vi "CreateTemporaryPath.vi"(8 "error in (no error)":errorcluster, 10 "InitalValue":T1, 11 "object in":refnum<class "Crypter.lvclass">) -> (0 "error out":errorcluster, 2 "ReferenceVariableOut":refnum<data-value>, 3 "object out":refnum<class "Crypter.lvclass">)   [LabVIEW 2018]
doc: "This VI creates a DVR reference for a variable."
uses:
  Crypter.lvclass
  C:/Users/Marco Preziani/Documents/Help_Crypting_repository/WebBrowser_Mgmt/WebBrowser_Mgmt.lvclass
  TemporaryPath.ctl
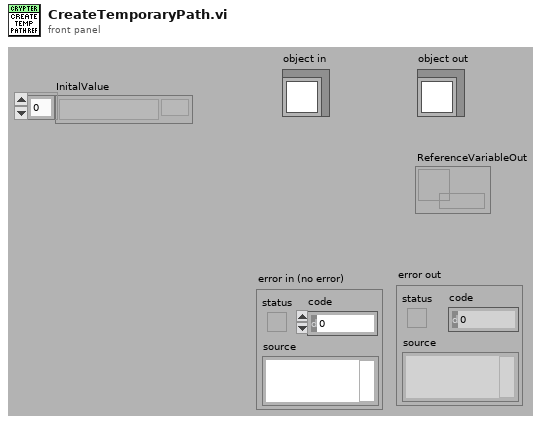
[diagram p1: front panel]
types:
  T1 = typedef "TemporaryPath.ctl" = path[]
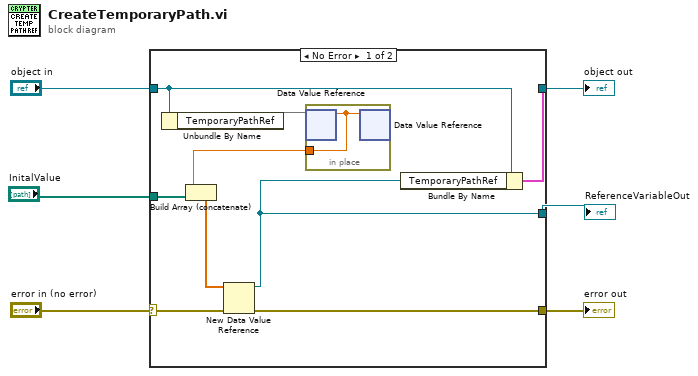
[diagram p0: block diagram]
diagram:
  n1 = case shown="No Error" "error in (no error)" {
    selector: "error in (no error)" -> [w15 w17]
    tunnel: [w13 w18] -> w6
    tunnel: [w14 w17] -> w5
    tunnel: "object in" -> [w10 w18]
    tunnel: "InitalValue" -> [w12 _]
    tunnel: [w11 _] -> w2
    frame No Error {
      n2 = Unbundle By Name(w10) -> ("TemporaryPathRef"=w8)
      n3 = in-place {
        in-place-border: [w16] -> w7
        n4 = in-place-dvr #1(w8) -> (w16:dbl)  [unwired: 1 out]
        n5 = in-place-dvr #1(w16) -> ()  [unwired: 2 out]
      }
      n6 = Build Array (concatenate)(w7, w12) -> (w9:dbl[])
      n7 = New Data Value Reference(data value=w9, error in=w15) -> (data value reference=w11:refnum<data-value>, error out=w14:errorcluster)
      n8 = Bundle By Name(cluster=w10, "TemporaryPathRef"=w11) -> (w13:cluster{})
    }
    frame Error {
    }
  }
  "error out" <- w5
  "object out" <- w6
  "ReferenceVariableOut" <- w2
